vi "CamPID.vi"() -> ()   [LabVIEW 2012]
uses:
  Autonomous_Routine_Global.vi
  <vilib>/addons/control/pid/pid.llb/PID (DBL).vi
  <vilib>/Rock Robotics/WPI/Joystick/WPI_JoystickGetSetRefNum.vi
  <vilib>/addons/control/pid/NI_PID_pid.lvlib
panel:
  in  "PID gains":T1={"proportional gain (Kc)"=1.0, "integral time (Ti, min)"=0.0, "derivative time (Td, min)"=0.0}
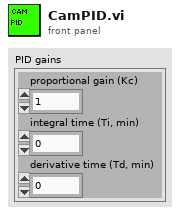
[diagram p1: front panel]
types:
  T1 = cluster{"proportional gain (Kc)":dbl, "integral time (Ti, min)":dbl, "derivative time (Td, min)":dbl}
  T2 = typedef "WPI_JoystickDevRef.ctl" = cluster{"Device":T3}
  T3 = typedef "WPI_JoystickDeviceEnum.ctl" = enum16{"USB 1", "USB 2", "USB 3", "USB 4", "Kinect 1", "Kinect 2"}
  T4 = cluster{"axis 1 (x)":dbl, "axis 2 (y)":dbl, "axis 3 (throttle)":dbl, "axis 4":dbl, "axis 5":dbl, "axis 6":dbl}
  T5 = typedef "WPI_MotorControlDeviceRef.ctl" = cluster{"DeviceStatus":errorcluster, "Type":enum16{"PWM", "CAN"}, "PWM":cluster{"Digital Module":T6, "PWM Channel":T7, "DeadBand":T8}, "CAN":cluster{"Device Number":u8, "Control Mode":T9, "Semaphore":T10, "Max Vout":dbl}, "Invert":bool, "TransformRef":T11, "InvTransformRef":T11}
  T6 = typedef "FPGA_TypedefDigitalModule.ctl" = enum16{"Digital Module 1", "Digital Module 2"}
  T7 = typedef "FPGA_DIOPWMChannel.ctl" = enum8{"PWM 1", "PWM 2", "PWM 3", "PWM 4", "PWM 5", "PWM 6", "PWM 7", "PWM 8", "PWM 9", "PWM 10", "Invalid"}
  T8 = typedef "WPI_PWMDeadband.ctl" = cluster{"Name":string, "maxPositivePwm":i32, "minPositivePwm":i32, "centerPwm":i32, "maxNegativePwm":i32, "minNegativePwm":i32, "angularRange":u16}
  T9 = typedef "WPI_CANJaguar_ControlMode.ctl" = enum8{"Percent VBus", "Current", "Speed", "Position", "Voltage"}
  T10 = typedef "Semaphore RefNum" = refnum<k1>
  T11 = typedef "WPI_PWMTransform_ConPane.ctl" = refnum<vi>
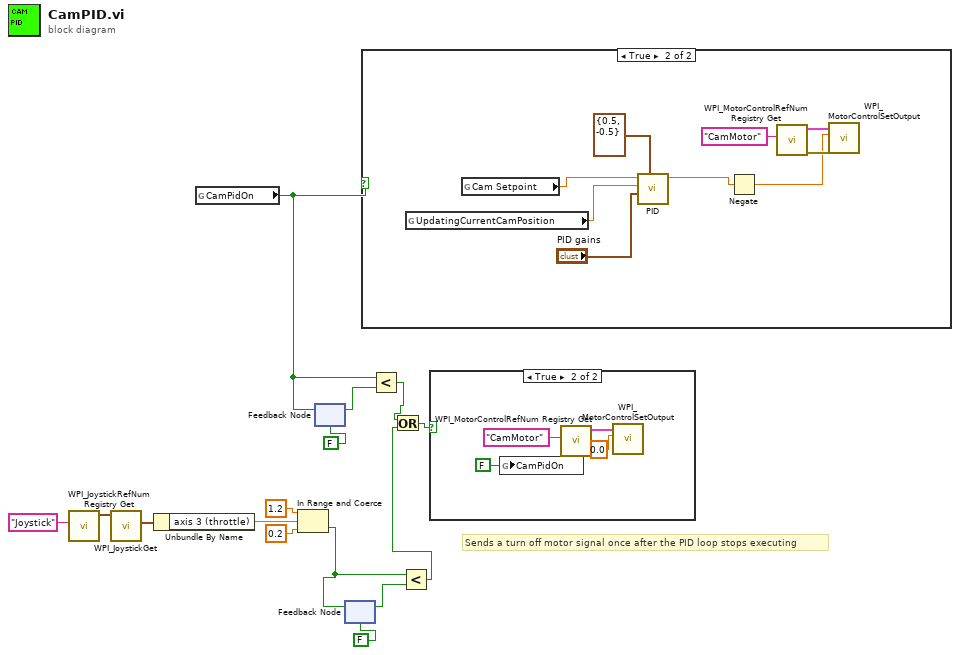
[diagram p0: block diagram]
diagram:
  # "Sends a turn off motor signal once after the PID loop stops executing"
  n1 = call <vilib>:"WPI_JoystickRefNum Registry Get.vi"("refnum name"="Joystick") -> ("JoystickDevRef"=w12:T2)  [unwired: 9 in, 1 out]
  n2 = call <vilib>:"WPI_JoystickGet.vi"("JoystickDevRef"=w12) -> ("Axes"=w10:T4)  [unwired: 4 in, 2 out]
  n3 = Unbundle By Name(w10) -> ("axis 3 (throttle)"=w9:dbl)
  n4 = global read "Autonomous_Routine_Global.vi" "CamPidOn"() -> (w13:bool)
  n5 = In Range and Coerce(upper limit=1.2, x=w9, lower limit=0.2 ("upper limit")) -> (In Range?=w4:bool)  [unwired: 1 out]
  n6 = feedback-in #1(w13) -> ()
  n7 = feedback #1(FALSE) -> (w15:bool)
  n8 = feedback #2(FALSE) -> (w5:bool)
  n9 = feedback-in #2(w4) -> ()
  n10 = case shown="True" w13 {
    frame False {
    }
    frame True {
      n11 = global read "Autonomous_Routine_Global.vi" "UpdatingCurrentCamPosition"() -> (w19:dbl)
      n12 = global read "Autonomous_Routine_Global.vi" "Cam Setpoint"() -> (w20:dbl)
      n13 = call-poly <vilib>:"PID.vi"("output range"=cluster{"output high":dbl, "output low":dbl} {"output high"=0.5, "output low"=-0.5}, "PID gains"="PID gains", "process variable"=w19, "setpoint"=w20) -> ("output"=w16:dbl)  [unwired: 6 in, 1 out]
      n14 = Negate(x=w16) -> (-x=w17:dbl)
      n15 = call <vilib>:"WPI_MotorControlRefNum Registry Get.vi"("refnum name"="CamMotor") -> ("error out"=w23:errorcluster, "MotorControlDevRef"=w22:T5)  [unwired: 9 in]
      n16 = call <vilib>:"WPI_MotorControlSetOutput.vi"("error in (no error)"=w23, "Output"=w17, "MotorControlDevRef"=w22) -> ()  [unwired: 6 in, 3 out]
    }
  }
  n17 = Less?(x=w13, y=w15) -> (x < y?=w2:bool)
  n18 = Less?(x=w4, y=w5) -> (x < y?=w1:bool)
  n19 = Or(x=w2, y=w1) -> (x .or. y?=w3:bool)
  n20 = case shown="True" w3 {
    frame False {
    }
    frame True {
      n21 = global write "Autonomous_Routine_Global.vi" "CamPidOn"(FALSE ("CamPidOn")) -> ()
      n22 = call <vilib>:"WPI_MotorControlRefNum Registry Get.vi"("refnum name"="CamMotor") -> ("MotorControlDevRef"=w27:T5)  [unwired: 9 in, 1 out]
      n23 = call <vilib>:"WPI_MotorControlSetOutput.vi"("Output"=0.0, "MotorControlDevRef"=w27) -> ()  [unwired: 7 in, 3 out]
    }
  }
